vi "Linear Equation.vi"(8 "Y-Int":dbl, 9 "Slope":dbl, 11 "X":dbl) -> (3 "Output":dbl)   [LabVIEW 2020]
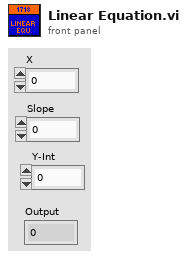
[diagram p1: front panel]
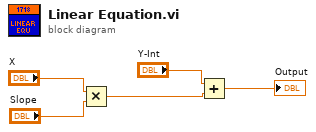
[diagram p0: block diagram]
diagram:
  n1 = Multiply(x="X", y="Slope") -> (x*y=w2:dbl)
  n2 = Add(x="Y-Int", y=w2) -> (x+y=→"Output":dbl)
